vi "Test Sweep API.vi"   [LabVIEW 2019]
uses:
  src/Instrument.Lockin/Instrument.Lockin.lvclass
  <vilib>/Analysis/1siggen.llb/Ramp Pattern by Samples.vi
  c3f68086-2c71-4676-baf4-799858c1ae09.vi
  1559a243-b7fb-4211-921b-e5aebecb1ff1.vi
  cdfe988a-f24c-4ea6-9edf-21cd4fa2a456.vi
  c3f68086-2c71-4676-baf4-799858c1ae09.vi/9e4911ce-1038-4ae1-8b68-6cf59a9e3e97.vi
  c3f68086-2c71-4676-baf4-799858c1ae09.vi/656972bd-b235-4613-8de2-4a0032e96b22.vi
  1559a243-b7fb-4211-921b-e5aebecb1ff1.vi/acc794b9-4b4e-4a75-948b-c17ed320e407.vi
  1559a243-b7fb-4211-921b-e5aebecb1ff1.vi/82c9d38d-8032-4cfa-9ba4-a496e9e113b5.vi
  cdfe988a-f24c-4ea6-9edf-21cd4fa2a456.vi/9c624f80-d7f2-42a2-84bb-ecc0ea5cd686.vi
  cdfe988a-f24c-4ea6-9edf-21cd4fa2a456.vi/104aa91d-93da-4d6e-88a0-70a19f8f9ea1.vi
  src/Instrument.Lockin/Private/Lockin.Remote Client.vi
  <vilib>/Analysis/NI_AALBase.lvlib
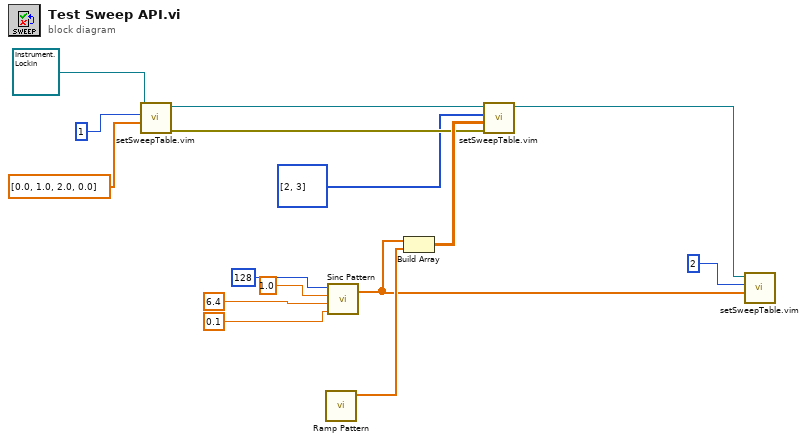
[diagram p0: block diagram]
diagram:
  n1 = call "setSweepTable.vim"("Table"=dbl[] [0.0, 1.0, 2.0, 0.0] ("Pattern"), "Channel"=1, "Instrument.Lockin in"=refnum<class "Instrument.Lockin.lvclass"> refnum) -> ("error out"=w5:errorcluster, "Instrument.Lockin out"=w2:refnum<class "Instrument.Lockin.lvclass">)  [unwired: 7 in]
  n2 = call-poly <vilib>:"Ramp Pattern.vi"() -> ("Ramp Pattern"=w14:dbl[])  [unwired: 10 in, 1 out]
  n3 = call <vilib>:"Sinc Pattern.vi"("delta t"=0.1, "delay"=6.4, "amplitude"=1.0, "samples"=128) -> ("Sinc Pattern"=w8:dbl[])  [unwired: 1 out]
  n4 = Build Array(w8, w14) -> (w15:dbl[][])
  n5 = call "setSweepTable.vim"("error in (no error)"=w5, "Table"=w15, "Channel"=i32[] [2, 3] ("Channel 2"), "Instrument.Lockin in"=w2) -> ("Instrument.Lockin out"=w3:refnum<class "Instrument.Lockin.lvclass">)  [unwired: 6 in, 1 out]
  n6 = call "setSweepTable.vim"("Table"=w8, "Channel"=2, "Instrument.Lockin in"=w3) -> ()  [unwired: 7 in, 2 out]
